vi "Send ERROR.vi"(8 "error in (no error)":errorcluster, 10 "Error Request":T1={"WAMP Error"={"Details"="{}", "ArgumentKw Payload"="", "Wamp error?"=FALSE, "Error URI"="", "Arguments Payload"=[]}, "Message Type"=0, "Request ID"=0} {"Message Type" items=["HELLO"=1, "WELCOME"=2, "ABORT"=3, "GOODBYE"=6, "ERROR"=8, "PUBLISH"=16, "PUBLISHED"=17, "SUBSCRIBE"=32, "SUBSCRIBED"=33, "UNSUBSCRIBE"=34, "UNSUBSCRIBED"=35, "EVENT"=36, "CALL"=48, "RESULT"=59, "REGISTER"=64, "REGISTERED"=65, "UNREGISTER"=66, "UNREGISTERED"=67, "INVOCATION"=68, "YIELD"=70]}, 11 "WAMP Client in":refnum<class "WAMP Client.lvclass">) -> (0 "error out":errorcluster, 3 "WAMP Client out":refnum<class "WAMP Client.lvclass">)   [LabVIEW 2020, in "wamplv.lvlib" / "WAMP Client.lvclass"]
uses:
  <vilib>/samangh/wamplv/WAMP Client/WAMP Client.lvclass
  <vilib>/samangh/wamplv/WAMP Client/TypeDef/Error Request.ctl
  <vilib>/samangh/wamplv/WAMP Client/TypeDef/WAMP Error Payload.ctl
  <vilib>/samangh/wamplv/WAMP Message Codes.ctl
  <vilib>/samangh/wamplv/WAMP Client/WAMP Client.lvclass/WAMP Client.ctl
  <vilib>/JDP Science/JSONtext/support/Format JSON Array Text.vi
  <vilib>/JDP Science/JSONtext/JSONtext.lvlib
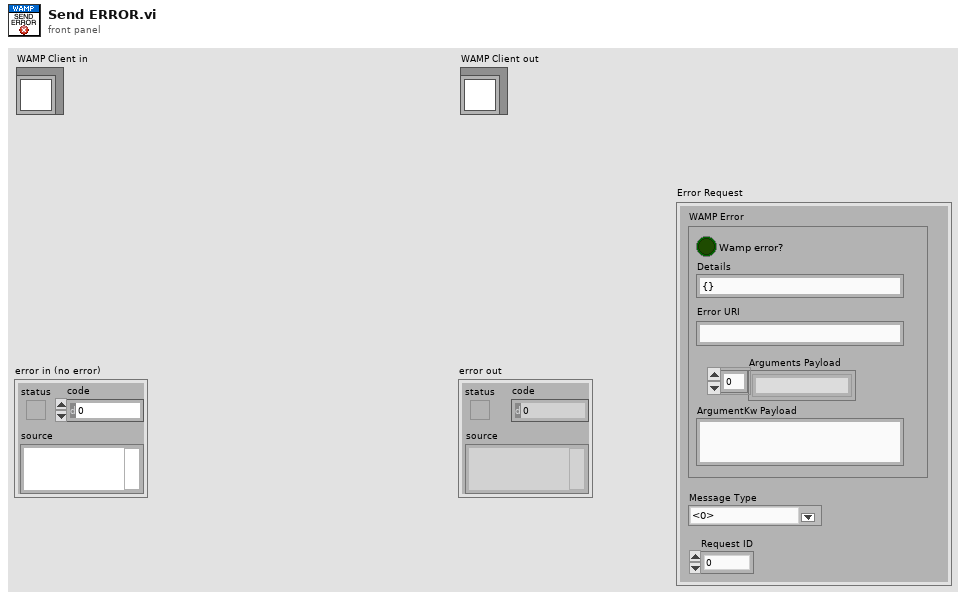
[diagram p1: front panel]
types:
  T1 = typedef "wamplv.lvlib/WAMP Client.lvclass/Error Request.ctl" = cluster{"WAMP Error":T2, "Message Type":T3, "Request ID":u64}
  T2 = typedef "wamplv.lvlib/WAMP Client.lvclass/WAMP Error Payload.ctl" = cluster{"Details":string, "ArgumentKw Payload":string, "Wamp error?":bool, "Error URI":string, "Arguments Payload":string[]}
  T3 = typedef "wamplv.lvlib/WAMP Client.lvclass/WAMP Message Codes.ctl" = u16
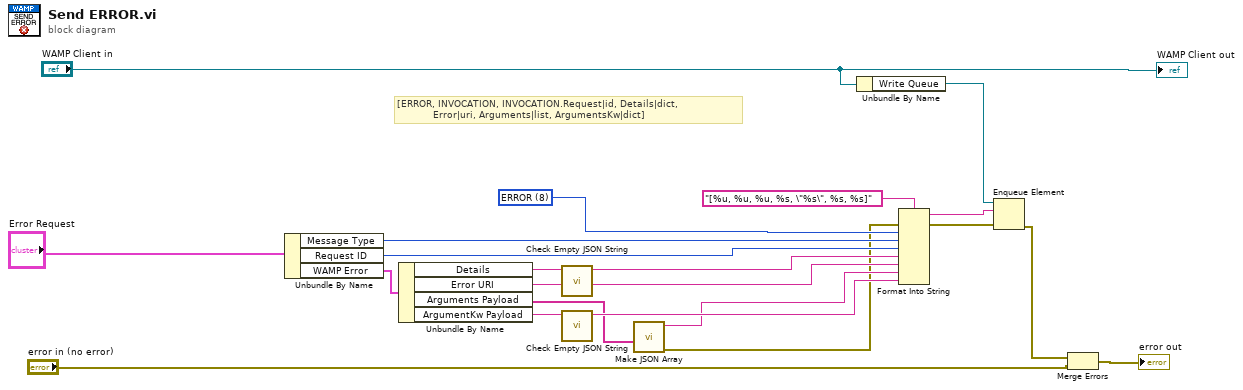
[diagram p0: block diagram]
diagram:
  w16 = T3 8 items=["HELLO"=1, "WELCOME"=2, "ABORT"=3, "GOODBYE"=6, "ERROR"=8, "PUBLISH"=16, "PUBLISHED"=17, "SUBSCRIBE"=32, "SUBSCRIBED"=33, "UNSUBSCRIBE"=34, "UNSUBSCRIBED"=35, "EVENT"=36, "CALL"=48, "RESULT"=59, "REGISTER"=64, "REGISTERED"=65, "UNREGISTER"=66, "UNREGISTERED"=67, "INVOCATION"=68, "YIELD"=70] ("Message Codes")
  # "[ERROR, INVOCATION, INVOCATION.Request|id, Details|dict,\n            Error|uri, Arguments|list, ArgumentsKw|dict]"
  n1 = Unbundle By Name("Error Request") -> ("Message Type"=w15:T3, "Request ID"=w14:u64, "WAMP Error"=w13:T2)
  n2 = Unbundle By Name(w13) -> ("Details"=w11:string, "Error URI"=w12:string, "Arguments Payload"=w3:string[], "ArgumentKw Payload"=w9:string)
  n3 = call <vilib>:"Check Empty JSON String.vi"("JSON"=w11) -> ("JSON"=w10:string)  [unwired: 10 in]
  n4 = call <vilib>:"Check Empty JSON String.vi"("JSON"=w9) -> ("JSON"=w8:string)  [unwired: 10 in]
  n5 = call <vilib>:"Make JSON Array.vi"("JSON Elements"=w3) -> ("error out"=w1:errorcluster, "<JSON>"=w2:string)  [unwired: 9 in]
  n6 = Unbundle By Name("WAMP Client in") -> ("Write Queue"=w17:refnum<queue>)
  n7 = Format Into String(format string="[%u, %u, %u, %s, \"%s\", %s, %s]" ("element"), error in=w1, w16, w15, w14, w10, w12, w2, w8) -> (resulting string=w19:string, error out=w18:errorcluster)  [unwired: 1 in]
  n8 = Enqueue Element(queue=w17, element=w19, error in (no error)=w18) -> (error out=w7:errorcluster)  [unwired: 1 in, 2 out]
  n9 = Merge Errors(w7, "error in (no error)") -> (→"error out":errorcluster)
  "WAMP Client out" <- "WAMP Client in"
